vi "Test Communication1.vi"(8 "error in":errorcluster, 11 "Channel out 2":u16) -> (0 "error out":errorcluster, 3 "Channel out":u16)   [LabVIEW 2025]
uses:
  a9163a1a-bf7f-4ec5-a553-ba6517dc0e79.vi
  PCAN2023/PCAN API.lvlib
  77574cea-78a9-48c4-8703-67bd64e21fec.vi
panel:
  in  "error out 2":errorcluster
  in  "x":bool
  out "Numeric":i32
  out "MessageBuffer out 2":T1 {"ID" format="%.0x"}
  out "Boolean 2":bool
  out "Boolean":bool
  out "MessageBuffer out":T1 {"ID" format="%.0x"}
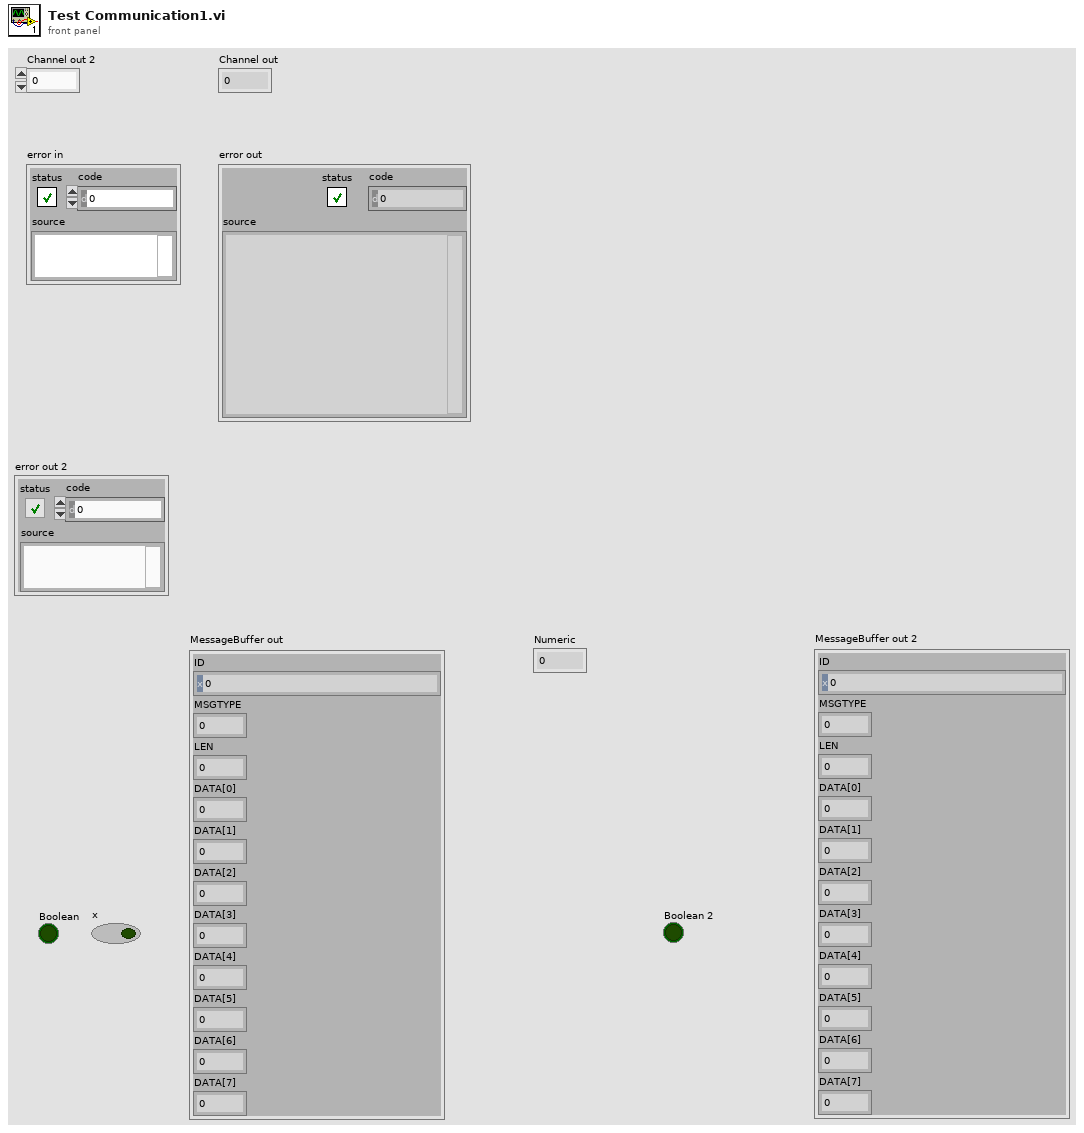
[diagram p1: front panel]
types:
  T1 = cluster{"ID":u32, "MSGTYPE":u8, "LEN":u8, "DATA[0]":u8, "DATA[1]":u8, "DATA[2]":u8, "DATA[3]":u8, "DATA[4]":u8, "DATA[5]":u8, "DATA[6]":u8, "DATA[7]":u8}
  T2 = cluster{"ID":u32, "MSGTYPE":u8, "DLC":u8, "DATA[0]":u8, "DATA[1]":u8, "DATA[2]":u8, "DATA[3]":u8, "DATA[4]":u8, "DATA[5]":u8, "DATA[6]":u8, "DATA[7]":u8, "DATA[8]":u8, "DATA[9]":u8, "DATA[10]":u8, "DATA[11]":u8, "DATA[12]":u8, "DATA[13]":u8, "DATA[14]":u8, "DATA[15]":u8, "DATA[16]":u8, "DATA[17]":u8, "DATA[18]":u8, "DATA[19]":u8, "DATA[20]":u8, "DATA[21]":u8, "DATA[22]":u8, "DATA[23]":u8, "DATA[24]":u8, "DATA[25]":u8, "DATA[26]":u8, "DATA[27]":u8, "DATA[28]":u8, "DATA[29]":u8, "DATA[30]":u8, "DATA[31]":u8, "DATA[32]":u8, "DATA[33]":u8, "DATA[34]":u8, "DATA[35]":u8, "DATA[36]":u8, "DATA[37]":u8, "DATA[38]":u8, "DATA[39]":u8, "DATA[40]":u8, "DATA[41]":u8, "DATA[42]":u8, "DATA[43]":u8, "DATA[44]":u8, "DATA[45]":u8, "DATA[46]":u8, "DATA[47]":u8, "DATA[48]":u8, "DATA[49]":u8, "DATA[50]":u8, "DATA[51]":u8, "DATA[52]":u8, "DATA[53]":u8, "DATA[54]":u8, "DATA[55]":u8, "DATA[56]":u8, "DATA[57]":u8, "DATA[58]":u8, "DATA[59]":u8, "DATA[60]":u8, "DATA[61]":u8, "DATA[62]":u8, "DATA[63]":u8}
  T3 = cluster{"ID":u32, "MSGTYPE":u8, "LEN":u8, "DATA[0]":u8, "DATA[1]":u8, "DATA[2]":u8, "DATA[3]":u8, "DATA[4]":u8, "DATA[5]":u8, "DATA[6]":u8, "DATA[7]":u8}[]
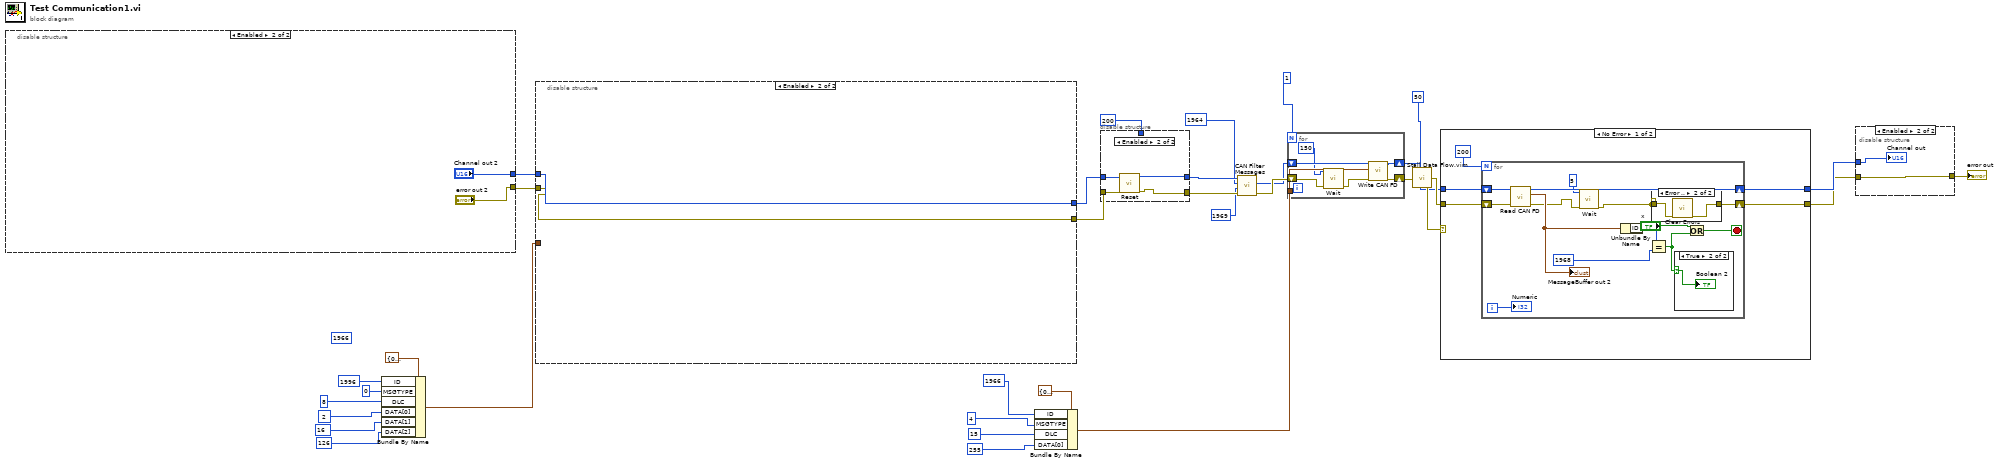
[diagram p0: block diagram]
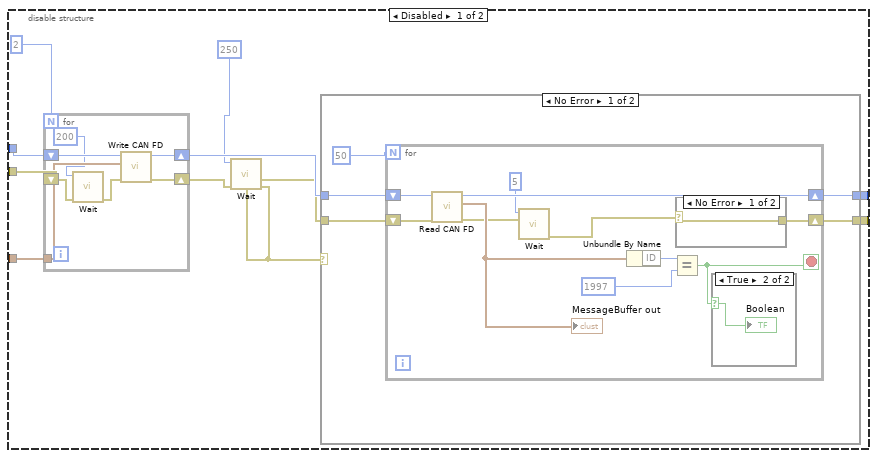
[diagram p2: hidden frame]
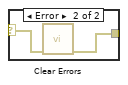
[diagram p3: hidden frame]
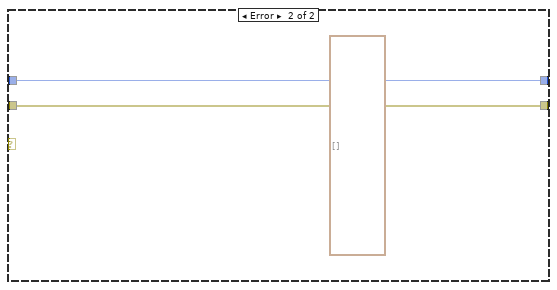
[diagram p5: hidden frame]
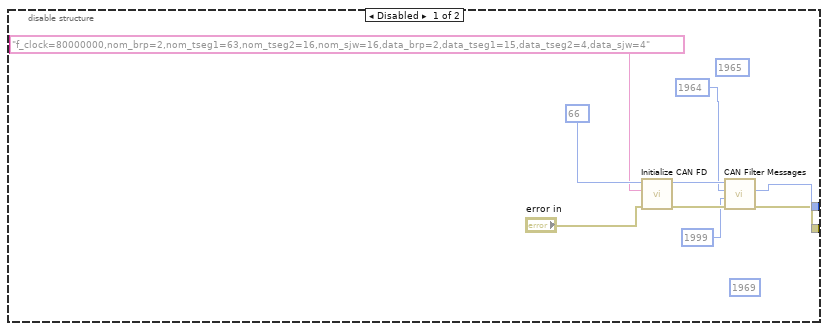
[diagram p6: hidden frame]
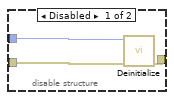
[diagram p7: hidden frame]
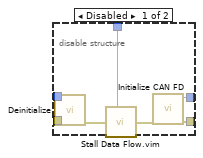
[diagram p8: hidden frame]
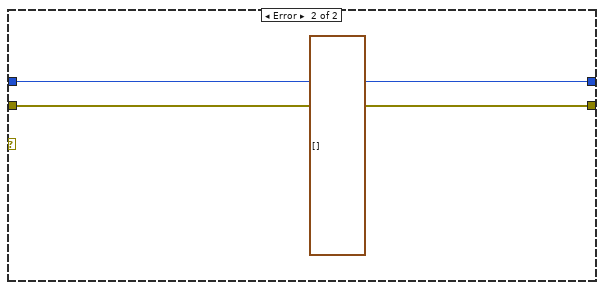
[diagram p11: hidden frame]
diagram:
  (unwired) u32 1966 ("ID")
  n1 = disable-structure shown="Enabled" {
    disable-tunnel: [w35 "Channel out 2"] -> w11
    disable-tunnel: [w34 "error out 2"] -> w10
    frame Disabled {
      (unwired) u32 1969 ("FromID")
      (unwired) u32 1965 ("FromID")
      n2 = call "Initialize CAN FD.vi"("error in"="error in", "BitrateFD"="f_clock=80000000,nom_brp=2,nom_tseg1=63,nom_tseg2=16,nom_sjw=16,data_brp=2,data_tseg1=15,data_tseg2=4,data_sjw=4", "Channel"=u16 66) -> ("error out"=w38:errorcluster, "Channel out"=w39:u16)  [unwired: 7 in]
      n3 = call "CAN Filter Messages.vi"("error in (no error)"=w38, "ToID"=u32 1999 ("FromID"), "FromID"=u32 1964, "Channel in"=w39) -> ("error out"=w34:errorcluster, "Channel out"=w35:u16)  [unwired: 5 in, 1 out]
    }
    frame Enabled {
    }
  }
  n4 = Bundle By Name(cluster=T2 {"ID"=0, "MSGTYPE"=0, "DLC"=0, "DATA[0]"=0, "DATA[1]"=0, "DATA[2]"=0, "DATA[3]"=0, "DATA[4]"=0, "DATA[5]"=0, "DATA[6]"=0, "DATA[7]"=0, "DATA[8]"=0, "DATA[9]"=0, "DATA[10]"=0, "DATA[11]"=0, "DATA[12]"=0, "DATA[13]"=0, "DATA[14]"=0, "DATA[15]"=0, "DATA[16]"=0, "DATA[17]"=0, "DATA[18]"=0, "DATA[19]"=0, "DATA[20]"=0, "DATA[21]"=0, "DATA[22]"=0, "DATA[23]"=0, "DATA[24]"=0, "DATA[25]"=0, "DATA[26]"=0, "DATA[27]"=0, "DATA[28]"=0, "DATA[29]"=0, "DATA[30]"=0, "DATA[31]"=0, "DATA[32]"=0, "DATA[33]"=0, "DATA[34]"=0, "DATA[35]"=0, "DATA[36]"=0, "DATA[37]"=0, "DATA[38]"=0, "DATA[39]"=0, "DATA[40]"=0, "DATA[41]"=0, "DATA[42]"=0, "DATA[43]"=0, "DATA[44]"=0, "DATA[45]"=0, "DATA[46]"=0, "DATA[47]"=0, "DATA[48]"=0, "DATA[49]"=0, "DATA[50]"=0, "DATA[51]"=0, "DATA[52]"=0, "DATA[53]"=0, "DATA[54]"=0, "DATA[55]"=0, "DATA[56]"=0, "DATA[57]"=0, "DATA[58]"=0, "DATA[59]"=0, "DATA[60]"=0, "DATA[61]"=0, "DATA[62]"=0, "DATA[63]"=0} ("MessageBuffer"), "ID"=u32 1996, "MSGTYPE"=u8 0, "DLC"=u8 8, "DATA[0]"=u8 2, "DATA[1]"=u8 16 ("DATA[0]"), "DATA[2]"=u8 126 ("DATA[0]")) -> (w32:T2)
  n5 = disable-structure shown="Enabled" {
    disable-tunnel: w32 -> [w54 _]
    disable-tunnel: w11 -> [w53 w85]
    disable-tunnel: w10 -> [w52 w84]
    disable-tunnel: [w49 w85] -> w9
    disable-tunnel: [w48 w84] -> w8
    frame Disabled {
      n6 = for {
        N: 2 -> [_]
        tunnel: w54 -> [w60]
        shift-right: [w59] -> w51
        shift-left: w53 -> [w61]
        shift-right: [w58] -> w47
        shift-left: w52 -> [w57]
        n7 = call "Wait.vi"("error in"=w57, "milliseconds to wait"=u32 200) -> ("error out"=w56:errorcluster)  [unwired: 9 in]
        n8 = call "Write CAN FD.vi"("error in (no error)"=w56, "MessageBuffer"=w60, "Channel"=w61) -> ("error out"=w58:errorcluster, "Channel out"=w59:u16)  [unwired: 7 in]
      }
      n9 = call "Wait.vi"("error in"=w47, "milliseconds to wait"=u32 250) -> ("error out"=w46:errorcluster)  [unwired: 9 in]
      n10 = case shown="No Error" w46 {
        tunnel: w51 -> [w66 w83]
        tunnel: w46 -> [w65 w82]
        tunnel: [w64 w83] -> w49
        tunnel: [w63 w82] -> w48
        frame No Error {
          n11 = for {
            N: 50 -> [_]
            shift-right: [w73] -> w64
            shift-left: w66 -> [w74]
            shift-right: [w75] -> w63
            shift-left: w65 -> [w72]
            stop <- w70 stop-if-true
            n12 = call "Read CAN FD.vi"("error in"=w72, "Channel"=w74) -> ("error out"=w69:errorcluster, "MessageBuffer out"=w71:T1, "Channel out"=w73:u16)  [unwired: 7 in]
            "MessageBuffer out" <- w71
            n13 = call "Wait.vi"("error in"=w69, "milliseconds to wait"=u32 5) -> ("error out"=w68:errorcluster)  [unwired: 9 in]
            n14 = Unbundle By Name(w71) -> ("ID"=w77:u32)
            n15 = Equal?(x=w77, y=u32 1997) -> (x = y?=w70:bool)
            n16 = case shown="No Error" w68 {
              selector: w68 -> [w78 w80]
              tunnel: [w78 w79] -> w75
              frame No Error {
              }
              frame Error {
                n17 = call <vilib>:"Clear Errors.vi"("error in (no error)"=w80) -> ("error out"=w79:errorcluster)  [unwired: 5 in, 1 out]
              }
            }
            n18 = case shown="True" w70 {
              selector: w70 -> [_ w81]
              frame False {
              }
              frame True {
                "Boolean" <- w81
              }
            }
          }
        }
        frame Error {
          (unwired) T3 []
        }
      }
    }
    frame Enabled {
    }
  }
  n19 = Bundle By Name(cluster=T2 {"ID"=0, "MSGTYPE"=0, "DLC"=0, "DATA[0]"=0, "DATA[1]"=0, "DATA[2]"=0, "DATA[3]"=0, "DATA[4]"=0, "DATA[5]"=0, "DATA[6]"=0, "DATA[7]"=0, "DATA[8]"=0, "DATA[9]"=0, "DATA[10]"=0, "DATA[11]"=0, "DATA[12]"=0, "DATA[13]"=0, "DATA[14]"=0, "DATA[15]"=0, "DATA[16]"=0, "DATA[17]"=0, "DATA[18]"=0, "DATA[19]"=0, "DATA[20]"=0, "DATA[21]"=0, "DATA[22]"=0, "DATA[23]"=0, "DATA[24]"=0, "DATA[25]"=0, "DATA[26]"=0, "DATA[27]"=0, "DATA[28]"=0, "DATA[29]"=0, "DATA[30]"=0, "DATA[31]"=0, "DATA[32]"=0, "DATA[33]"=0, "DATA[34]"=0, "DATA[35]"=0, "DATA[36]"=0, "DATA[37]"=0, "DATA[38]"=0, "DATA[39]"=0, "DATA[40]"=0, "DATA[41]"=0, "DATA[42]"=0, "DATA[43]"=0, "DATA[44]"=0, "DATA[45]"=0, "DATA[46]"=0, "DATA[47]"=0, "DATA[48]"=0, "DATA[49]"=0, "DATA[50]"=0, "DATA[51]"=0, "DATA[52]"=0, "DATA[53]"=0, "DATA[54]"=0, "DATA[55]"=0, "DATA[56]"=0, "DATA[57]"=0, "DATA[58]"=0, "DATA[59]"=0, "DATA[60]"=0, "DATA[61]"=0, "DATA[62]"=0, "DATA[63]"=0} ("MessageBuffer"), "ID"=u32 1966, "MSGTYPE"=u8 4, "DLC"=u8 15, "DATA[0]"=u8 255) -> (w20:T2)
  n20 = disable-structure shown="Enabled" {
    disable-tunnel: w9 -> [w92 w96]
    disable-tunnel: w8 -> [w91 w95]
    disable-tunnel: [w90 w94] -> w7
    disable-tunnel: [w88 w93] -> w6
    disable-tunnel: u32 200 ("milliseconds to wait") -> [w86 _]
    frame Disabled {
      n21 = call "Deinitialize.vi"("error in"=w91, "Channel"=w92) -> ("error out"=w89:errorcluster)  [unwired: 9 in]
      n22 = call "Stall Data Flow.vim"("value in"=w89, "milliseconds to wait"=w86) -> ("value out"=w87:errorcluster)  [unwired: 1 out]
      n23 = call "Initialize CAN FD.vi"("error in"=w87) -> ("error out"=w88:errorcluster, "Channel out"=w90:u16)  [unwired: 9 in]
    }
    frame Enabled {
      n24 = call "Reset.vi"("error in"=w95, "Channel"=w96) -> ("error out"=w93:errorcluster, "Channel out"=w94:u16)  [unwired: 8 in]
    }
  }
  n25 = call "CAN Filter Messages.vi"("error in (no error)"=w6, "ToID"=u32 1969 ("FromID"), "FromID"=u32 1964, "Channel in"=w7) -> ("error out"=w5:errorcluster, "Channel out"=w4:u16)  [unwired: 5 in, 1 out]
  n26 = for {
    N: 1 -> [_]
    tunnel: w20 -> [w102]
    shift-right: [w101] -> w17
    shift-left: w4 -> [w103]
    shift-right: [w100] -> w16
    shift-left: w5 -> [w98]
    n27 = call "Wait.vi"("error in"=w98, "milliseconds to wait"=u32 150) -> ("error out"=w97:errorcluster)  [unwired: 9 in]
    n28 = call "Write CAN FD.vi"("error in (no error)"=w97, "MessageBuffer"=w102, "Channel"=w103) -> ("error out"=w100:errorcluster, "Channel out"=w101:u16)  [unwired: 7 in]
  }
  n29 = call "Stall Data Flow.vim"("value in"=w16, "milliseconds to wait"=u32 50) -> ("value out"=w18:errorcluster)  [unwired: 1 out]
  n30 = case shown="No Error" w18 {
    tunnel: w17 -> [w108 w128]
    tunnel: w18 -> [w107 w127]
    tunnel: [w106 w128] -> w15
    tunnel: [w105 w127] -> w14
    frame No Error {
      n31 = for {
        N: 200 -> [_]
        shift-right: [w119] -> w106
        shift-left: w108 -> [w120]
        shift-right: [w121] -> w105
        shift-left: w107 -> [w118]
        i -> [w116]
        stop <- w113 stop-if-true
        n32 = call "Read CAN FD.vi"("error in"=w118, "Channel"=w120) -> ("error out"=w111:errorcluster, "MessageBuffer out"=w112:T1, "Channel out"=w119:u16)  [unwired: 7 in]
        "MessageBuffer out 2" <- w112
        n33 = call "Wait.vi"("error in"=w111, "milliseconds to wait"=u32 5) -> ("error out"=w110:errorcluster)  [unwired: 9 in]
        n34 = Unbundle By Name(w112) -> ("ID"=w117:u32)
        n35 = Equal?(x=w117, y=u32 1968) -> (x = y?=w115:bool)
        n36 = case shown="Error .." w110 {
          selector: w110 -> [w123 w125]
          tunnel: w110 -> [_ _]
          tunnel: [w123 w124] -> w121
          frame No Error {
          }
          frame Error {
            n37 = call <vilib>:"Clear Errors.vi"("error in (no error)"=w125) -> ("error out"=w124:errorcluster)  [unwired: 5 in, 1 out]
          }
        }
        n38 = case shown="True" w115 {
          selector: w115 -> [_ w126]
          frame False {
          }
          frame True {
            "Boolean 2" <- w126
          }
        }
        n39 = Or(x="x", y=w115) -> (x .or. y?=w113:bool)
        "Numeric" <- w116
      }
    }
    frame Error {
      (unwired) T3 []
    }
  }
  n40 = disable-structure shown="Enabled" {
    disable-tunnel: [w131 w133] -> w27
    disable-tunnel: w15 -> [w130 w132]
    disable-tunnel: w14 -> [w129 w133]
    frame Disabled {
      n41 = call "Deinitialize.vi"("error in"=w129, "Channel"=w130) -> ("error out"=w131:errorcluster)  [unwired: 9 in]
    }
    frame Enabled {
      "Channel out" <- w132
    }
  }
  "error out" <- w27
